vi "Hardware_auto_detection_test.vi"() -> ()   [LabVIEW 2018]
uses:
  SubVi's/Controls/CTL_VISA_port_Descr.-Name.ctl
  <vilib>/Instr/_visa.llb/VISA Configure Serial Port (Instr).vi
  Common_Resources.lvlib
panel:
  in  "COM-ports selector":i32(listbox)
  out "Detected COM ports":T1[](array[typedef])
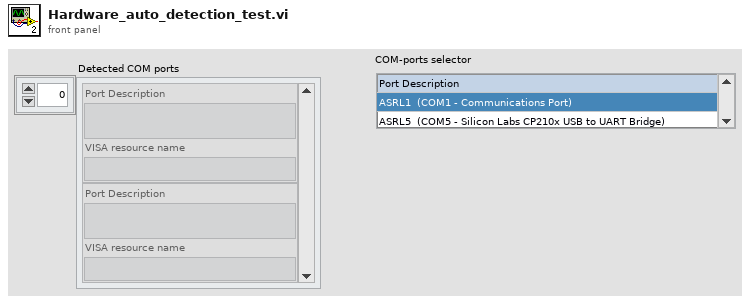
[diagram p1: front panel]
types:
  T1 = typedef "Common_Resources.lvlib/CTL_VISA_port_Descr.-Name.ctl" = cluster{"Port Description":string, "VISA resource name":string}
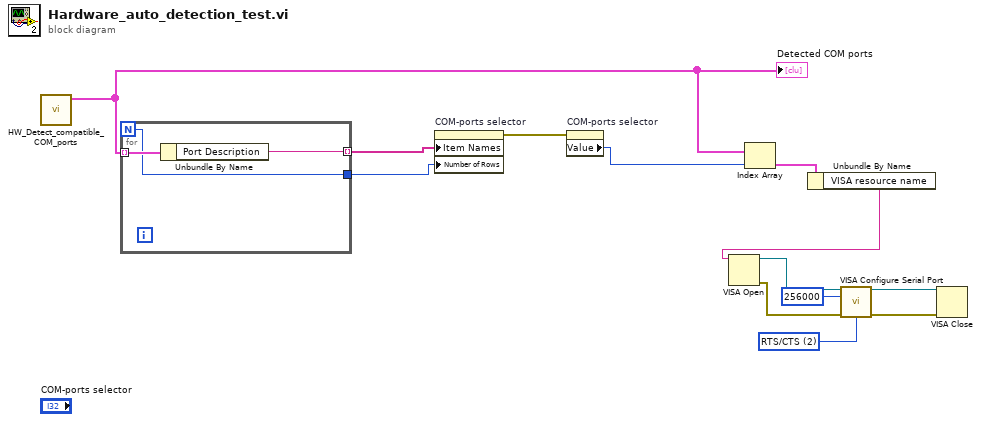
[diagram p0: block diagram]
diagram:
  w4 = u16 2 items=["None", "XON/XOFF", "RTS/CTS", "XON/XOFF & RTS/CTS", "DTR/DSR", "XON/XOFF & DTR/DSR"] ("flow control (0:none)")
  n1 = call "HW_Detect_compatible_COM_ports.vi"() -> ("Detected COM ports"=w10:T1[])  [unwired: 2 in, 3 out]
  "Detected COM ports" <- w10
  n2 = for {
    N -> [w14]
    tunnel: w10 -> [w16] mode=indexing
    tunnel: [w15] -> w13 mode=indexing
    tunnel: [w14] -> w12
    n3 = Unbundle By Name(w16) -> ("Port Description"=w15:string)
  }
  n4 = property on="COM-ports selector" class="LstBox (strict)"("Item Names"=w13, "Number of Rows"=w12) -> (error out=w11:errorcluster)  [unwired: 2 in, 1 out]
  n5 = property on="COM-ports selector" class="LstBox (strict)"(error in=w11) -> ("Value"=w9:i32)  [unwired: 1 in, 2 out]
  n6 = Index Array(array=w10, index=w9) -> (element=w8:T1)
  n7 = Unbundle By Name(w8) -> ("VISA resource name"=w7:string)
  n8 = VISA Open(VISA resource name=w7) -> (VISA resource name=w6:refnum<visa-resource-name>, error out=w2:errorcluster)  [unwired: 4 in]
  n9 = call-poly "VISA Configure Serial Port"("VISA resource name"=w6, "baud rate (9600)"=u32 256000, "error in (no error)"=w2, "flow control (0:none)"=w4) -> ("VISA resource name out"=w3:refnum<visa-resource-name>, "error out"=w1:errorcluster)  [unwired: 10 in]
  n10 = VISA Close(VISA resource name=w3, error in (no error)=w1) -> ()  [unwired: 1 out]
